vi "Configure Basic Input Output Phase.vi"(6 "Append Traces (T: Enable)":bool=TRUE, 7 "FFT Lines (0: fftl32k)":i32(ring) items=["fftl32k", "fftl16k", "fftl8k", "fftl4k", "fftl2k", "fftl1k", "fftl512", "fftl256"], 8 "error in (no error)":errorcluster, 9 "Selection Type (0: mPhase)":i32(ring) items=["mPhase", "mPhaseGroupDelay"], 10 "Waveform (0: wcChirp)":i32(ring) items=["wcChirp", "wcChirpPnk"], 11 "VISA resource name":refnum<visa-resource-name>) -> (0 "error out":errorcluster, 3 "VISA resource name out":refnum<visa-resource-name>)   [LabVIEW 2014, in "Stanford Research SR1.lvlib"]
doc: "Configures the basic attributes of the Input Output Phase Quick Measurement."
uses:
  Stanford Research SR1.lvlib
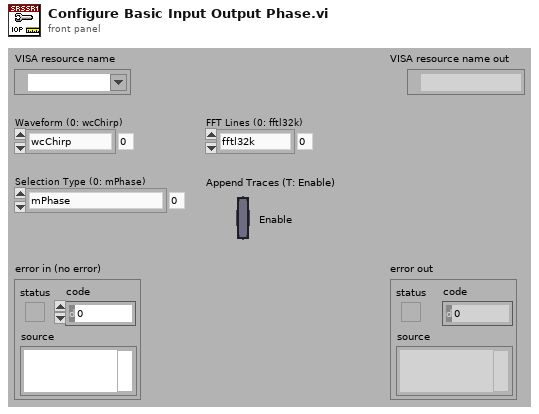
[diagram p1: front panel]
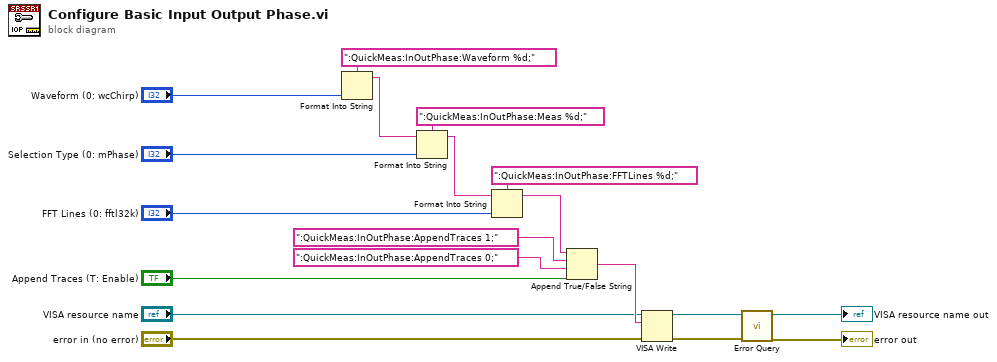
[diagram p0: block diagram]
diagram:
  n1 = Format Into String(format string=":QuickMeas:InOutPhase:Waveform %d;", "Waveform (0: wcChirp)") -> (resulting string=w17:string)  [unwired: 2 in, 1 out]
  n2 = Format Into String(format string=":QuickMeas:InOutPhase:Meas %d;", initial string=w17, "Selection Type (0: mPhase)") -> (resulting string=w14:string)  [unwired: 1 in, 1 out]
  n3 = Format Into String(format string=":QuickMeas:InOutPhase:FFTLines %d;", initial string=w14, "FFT Lines (0: fftl32k)") -> (resulting string=w11:string)  [unwired: 1 in, 1 out]
  n4 = Append True/False String(1:"Append Traces (T: Enable)", 2:":QuickMeas:InOutPhase:AppendTraces 0;", 3:":QuickMeas:InOutPhase:AppendTraces 1;", 4:w11) -> (0:w7:string)
  n5 = VISA Write(VISA resource name="VISA resource name", write buffer=w7, error in (no error)="error in (no error)") -> (VISA resource name out=w4:refnum<visa-resource-name>, error out=w3:errorcluster)  [unwired: 1 out]
  n6 = call "Error Query.vi"("error in (no error)"=w3, "VISA resource name"=w4) -> ("error out"=→"error out":errorcluster, "VISA resource name out"=→"VISA resource name out":refnum<visa-resource-name>)  [unwired: 6 in, 2 out]
